vi "ADIS16470 Loop Custom.vi"(8 "error in":errorcluster) -> ()   [LabVIEW 2018]
uses:
  Typedef/ADIS16470 Hardware Configuration.ctl
  <vilib>/Rock Robotics/WPI/SPI/WPI_SPIMode.ctl
  <vilib>/Rock Robotics/SystemInterfaces/DIO/FPGA_DIOChannel.ctl
  <vilib>/Rock Robotics/SystemInterfaces/spilib/spi_bus.ctl
  Typedef/ADIS16470 Process.ctl
  Typedef/ADIS16470 Device Reference.ctl
  Typedef/ADIS16470 Data.ctl
  Typedef/ADIS16470 Status.ctl
  Typedef/ADIS16470 Command Type.ctl
  <vilib>/Rock Robotics/WPI/SPI/WPI_SPIDevRef.ctl
  <vilib>/Rock Robotics/WPI/Interrupt/WPI_InterruptRef.ctl
  <vilib>/Rock Robotics/SystemInterfaces/Interrupt/FPGA_InterruptIndex.ctl
  <vilib>/Rock Robotics/WPI/Encoder/WPI_EncoderDevRef.ctl
  <vilib>/Rock Robotics/SystemInterfaces/Encoder/FPGA_EncoderIdx.ctl
  <vilib>/Rock Robotics/SystemInterfaces/Counter/FPGA_CounterCtrSystemIndex.ctl
  <vilib>/Rock Robotics/WPI/Encoder/WPI_EncoderType.ctl
  <vilib>/Rock Robotics/SystemInterfaces/NetworkCommunication/NetComm_UsageReport_ResourceType.ctl
  Typedef/ADIS16470 Register.ctl
  <vilib>/Rock Robotics/WPI/Counter/WPI_CounterDigitalInputToDigitalSource.vi
  <vilib>/Rock Robotics/SystemInterfaces/CounterEncoderSourceConvertion/FPGA_CounterEncoderSourceConvertionLVSourceTypeToFPGAType.vi
  <vilib>/Rock Robotics/WPI/Interrupt/WPI_InterruptCache.vi
  <vilib>/Rock Robotics/SystemInterfaces/Interrupt/FPGA_InterruptWriteConfiguration.vi
  <vilib>/Rock Robotics/SystemInterfaces/Interrupt/FPGA_WaitOnInterrupt.vi
  <vilib>/Rock Robotics/WPI/Utilities/WPI_UtilitiesTimebaseConstants.vi
  <vilib>/Rock Robotics/SystemInterfaces/Interrupt/FPGA_InterruptReadTimestamp.vi
panel:
  in  "Sychronous Process VI":T1
  in  "Hardware Config":T2={"SPI Clock Rate (Hz)"=2000000.0, "IMU SPI Mode (3)"=enum."Mode 3 (Clk Idle High,Sample on Trailing)", "IMU Reset Pin"=enum."SPI Port CS2", "IMU SPI Bus"=enum."SPI On-Board, CS0", "IMU Data Ready Pin"=enum."SPI Port CS1"}
  out "Waveform Chart":dbl(graph)
  out "Offset Bias":i16[](array[numeric])
  out "xAngle":dbl
  out "yAngle":dbl
  out "Data":dbl[](array[numeric])
  out "Counter":u16
  # "x"
  # "y"
  # "z"
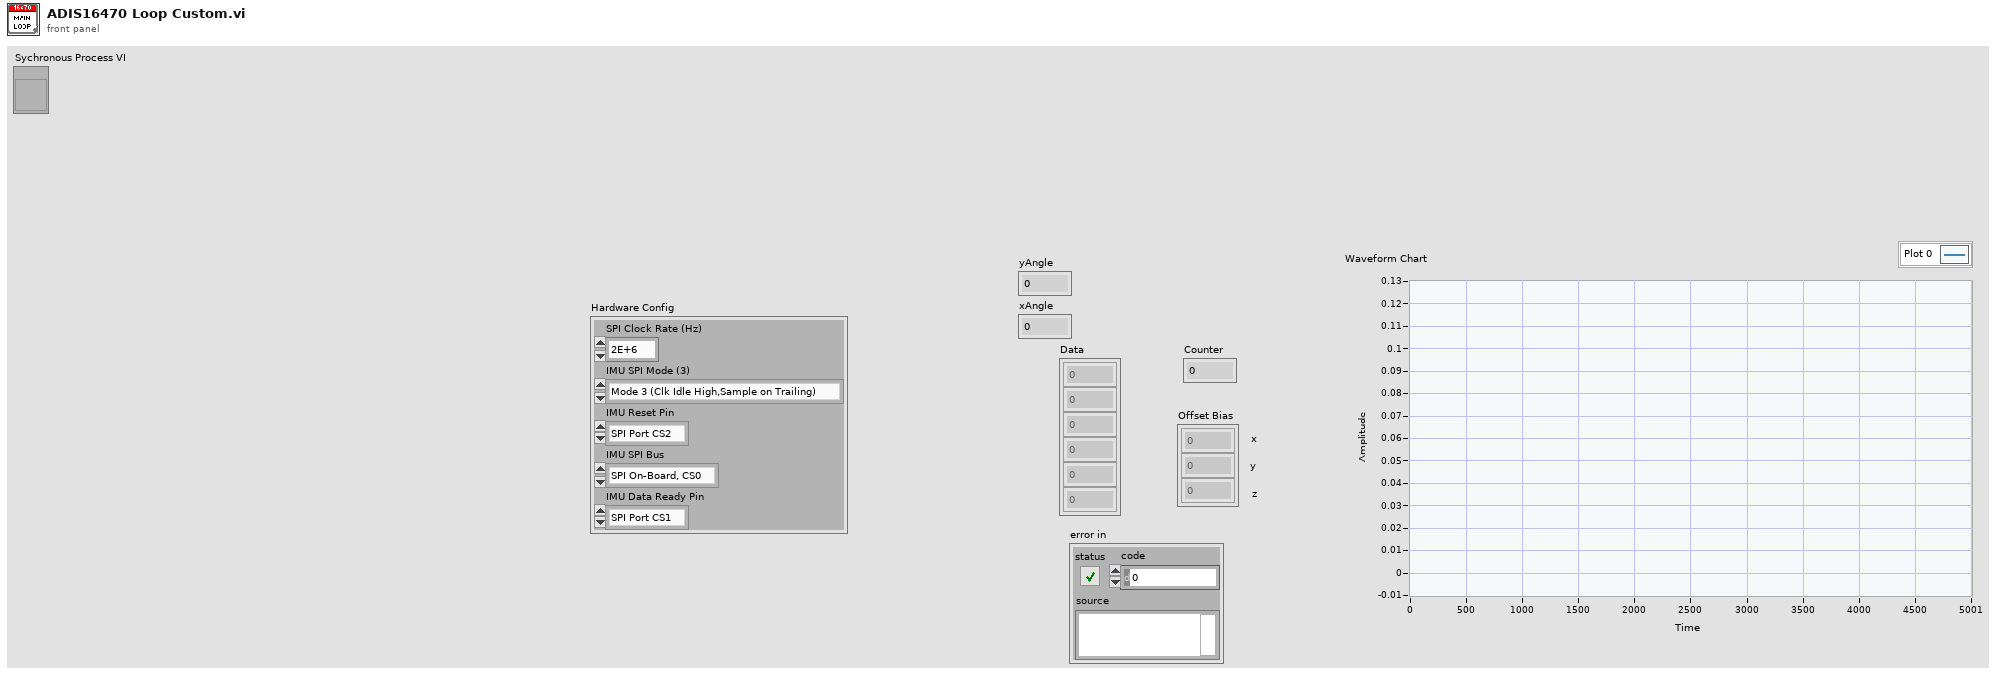
[diagram p1: front panel]
types:
  T1 = typedef "ADIS16470 Process.ctl" = refnum<vi>
  T2 = typedef "ADIS16470 Hardware Configuration.ctl" = cluster{"SPI Clock Rate (Hz)":dbl, "IMU SPI Mode (3)":T3, "IMU Reset Pin":T4, "IMU SPI Bus":T5, "IMU Data Ready Pin":T4}
  T3 = typedef "WPI_SPIMode.ctl" = enum16{"Mode 0 (Clk Idle Low,Sample on Leading)", "Mode 1 (Clk Idle Low,Sample on Trailing)", "Mode 2 (Clk Idle High,Sample on Leading)", "Mode 3 (Clk Idle High,Sample on Trailing)"}
  T4 = typedef "FPGA_DIOChannel.ctl" = enum8{"DIO 0", "DIO 1", "DIO 2", "DIO 3", "DIO 4", "DIO 5", "DIO 6", "DIO 7", "DIO 8", "DIO 9", "DIO MXP 0", "DIO MXP 1", "DIO MXP 2", "DIO MXP 3", "DIO MXP 4", "DIO MXP 5", "DIO MXP 6", "DIO MXP 7", "DIO MXP 8", "DIO MXP 9", "DIO MXP 10", "DIO MXP 11", "DIO MXP 12", "DIO MXP 13", "DIO MXP 14", "DIO MXP 15", "SPI Port CS1", "SPI Port CS2", "SPI Port CS3", "SPI Port MISO", "SPI Port MOSI", "Invalid"}
  T5 = typedef "spi_bus.ctl" = enum16{"SPI On-Board, CS0", "SPI On-Board, CS1", "SPI On-Board, CS2", "SPI On-Board, CS3", "SPI MXP", "Invalid"}
  T6 = typedef "NetComm_UsageReport_ResourceType.ctl" = enum8{"Controller", "Module", "Language", "CANPlugin", "Accelerometer", "ADXL345", "AnalogChannel", "AnalogTrigger", "AnalogTriggerOutput", "CANJaguar", "Compressor", "Counter", "Dashboard", "DigitalInput", "DigitalOutput", "DriverStationCIO", "DriverStationEIO", "DriverStationLCD", "Encoder", "GearTooth", "Gyro", "I2C", "Framework", "Jaguar", "Joystick", "Kinect", "KinectStick", "PIDController", "Preferences", "PWM", "Relay", "RobotDrive", "SerialPort", "Servo", "Solenoid", "SPI", "Task", "Ultrasonic", "Victor", "Button", "Command", "AxisCamera", "PCVideoServer", "SmartDashboard", "Talon", "HiTechnicColorSensor", "HiTechnicAccel", "HiTechnicCompass", "SRF08", "AnalogOutput", "Victor SP", "Talon SRX", "CAN Talon SRX", "ADXL362 Accel", "ADXRS450 Gyro", "Rev SPARK", "Mindsensors SD540", "Digital Filter", "ADIS16448", "PDP", "PCM", "PigeonIMU", "Nidec Brushless", "CTRE CANifier", "CTRE Future 0", "CTRE Future 1", "CTRE Future 2", "CTRE Future 3", "CTRE Future 4", "CTRE Future 5", "CTRE Future 6", "Linear Filter", "Xbox Controller", "USB Camera", "NavX", "Pixy", "Pixy2", "ScanseSweep", "Shuffleboard", "CAN", "Digilent DMC60", "PWM Victor SPX", "Rev SPARK MAX PWM", "Rev SPARK MAX CAN", "ADIS16470"}
  T7 = typedef "ADIS16470 Command Type.ctl" = enum16{"None", "Reset"}
  T8 = typedef "ADIS16470 Device Reference.ctl" = cluster{"DevStatus":errorcluster, "Hardware Config":T2, "End Calibration":refnum<notifier>, "Calibration Complete":refnum<notifier>, "Data FIFO":refnum<k33>, "Status FIFO":refnum<k33>, "Last Value Reference":refnum<data-value>, "Sychronous Process VI":T1, "Cmd FIFO":refnum<k33>}
  T9 = typedef "ADIS16470 Data.ctl" = cluster{"Yaw":dbl, "Timestamp":dbl, "Timestamp Delta":dbl, "Sample Count":u16}
  T10 = typedef "ADIS16470 Status.ctl" = cluster{"Calibrated?":bool}
  T11 = typedef "WPI_SPIDevRef.ctl" = cluster{"DevStatus":errorcluster, "Handle":i32, "SPI Bus":T5}
  T12 = typedef "WPI_InterruptRef.ctl" = cluster{"DevStatus":errorcluster, "InterruptIndex":T13}
  T13 = typedef "FPGA_InterruptIndex.ctl" = enum8{"0", "1", "2", "3", "4", "5", "6", "7", "Invalid"}
  T14 = typedef "WPI_EncoderDevRef.ctl" = cluster{"DevStatus":errorcluster, "EncoderIndex":T15, "CounterIndex":T16, "DistancePerCount":dbl, "Decoding Type":T17}
  T15 = typedef "FPGA_EncoderIdx.ctl" = enum8{"Enc 0", "Enc 1", "Enc 2", "Enc 3", "Enc 4", "Enc 5", "Enc 6", "Enc 7", "Invalid"}
  T16 = typedef "FPGA_CounterCtrSystemIndex.ctl" = enum8{"Ctr 0", "Ctr 1", "Ctr 2", "Ctr 3", "Ctr 4", "Ctr 5", "Ctr 6", "Ctr 7", "Invalid"}
  T17 = typedef "WPI_EncoderType.ctl" = enum16{"1x", "2x", "4x"}
  T18 = cluster{"ADIS16470DevRef":T8, "SPIDevRef":T11, "InterruptRef":T12, "Sensor to Robot Rotation":dbl[][], "Yaw":dbl, "Data Counter":u16, "First Run":bool, "TimeStamp Prev":dbl, "Time Delta":dbl, "Encoder Right":T14, "Encoder Left":T14, "Encoder Data":cluster{"Left Distance":dbl, "Right Distance":dbl}}
  T19 = typedef "ADIS16470 Register.ctl" = u8
  T20 = typedef "WPI_DigitalOutputDevRef.ctl" = cluster{"DIO Channel":T4, "DevStatus":errorcluster}
  T21 = typedef "WPI_DigitalInputDevRef.ctl" = cluster{"DevStatus":errorcluster, "DIO Channel":T4}
  T22 = typedef "FPGA_CounterEncoderSourceConvertionLVSourceType.ctl" = cluster{"DevStatus":errorcluster, "AnalogTriggerMode?":bool, "DigitalMode":cluster{"DIO Channel":T23}, "AnalogTriggerMode":cluster{"AnalogTriggerIndex":T24, "OutputType":T25}}
  T23 = typedef "FPGA_DIODigitalSourceChannel.ctl" = enum8{"DIO 0", "DIO 1", "DIO 2", "DIO 3", "DIO 4", "DIO 5", "DIO 6", "DIO 7", "DIO 8", "DIO 9", "DIO MXP 0", "DIO MXP 1", "DIO MXP 2", "DIO MXP 3", "DIO MXP 4", "DIO MXP 5", "DIO MXP 6", "DIO MXP 7", "DIO MXP 8", "DIO MXP 9", "DIO MXP 10", "DIO MXP 11", "DIO MXP 12", "DIO MXP 13", "DIO MXP 14", "DIO MXP 15", "SPI Port CS1", "SPI Port CS2", "SPI Port CS3", "SPI Port MISO", "SPI Port MOSI", "Disabled"}
  T24 = typedef "FPGA_AnalogTriggerIndex.ctl" = enum8{"Trig 0", "Trig 1", "Trig 2", "Trig 3", "Trig 4", "Trig 5", "Trig 6", "Trig 7", "Invalid"}
  T25 = typedef "FPGA_AnalogTriggerOutType.ctl" = enum16{"InWindow", "TriggerState", "Rising", "Falling"}
  T26 = cluster{"Left Distance":dbl, "Right Distance":dbl}
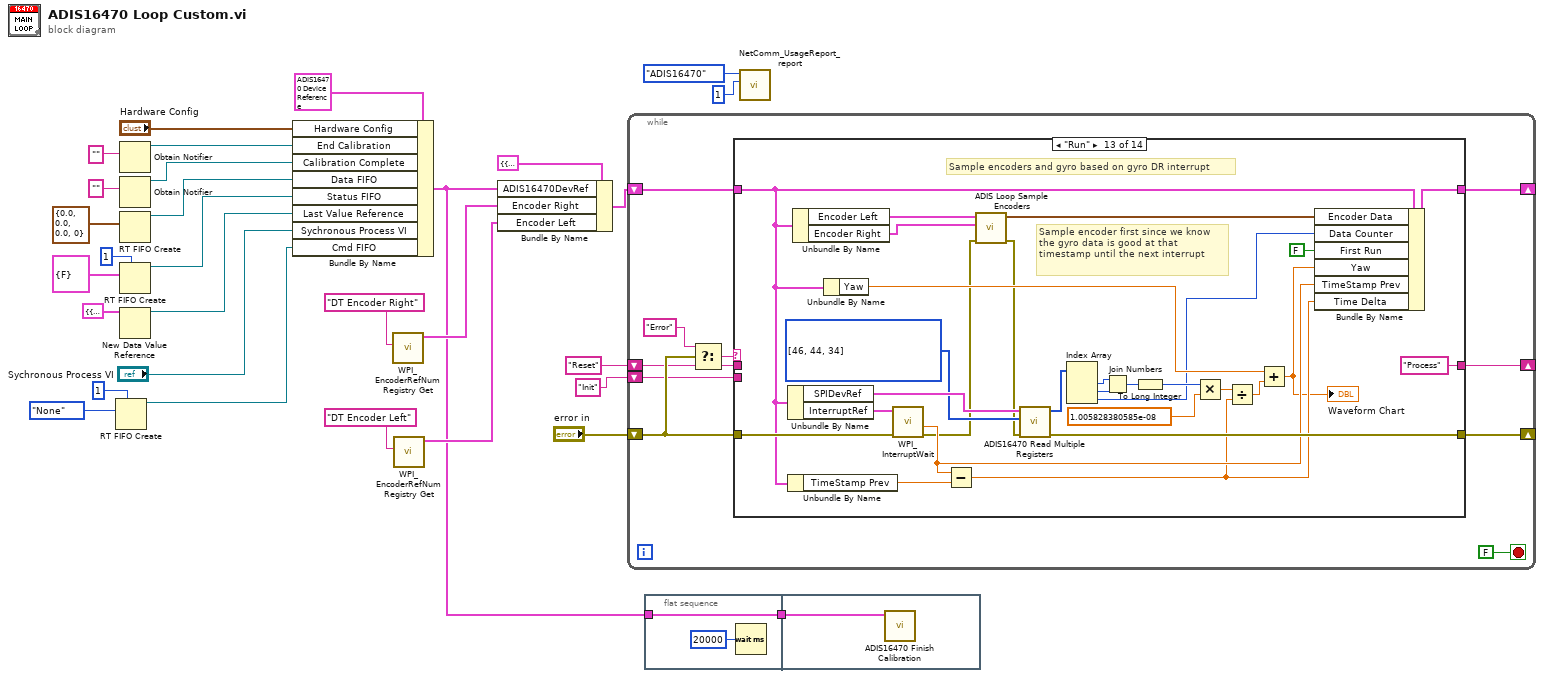
[diagram p0: block diagram]
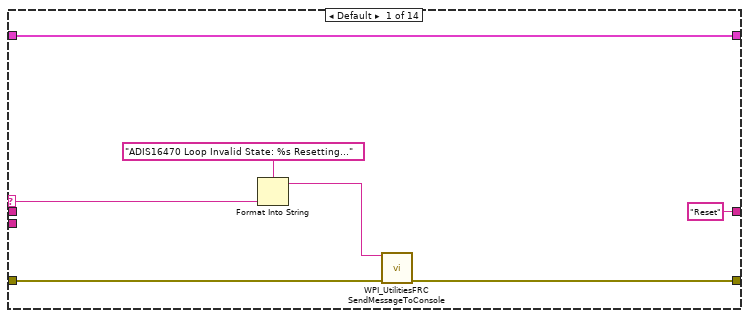
[diagram p2: hidden frame]
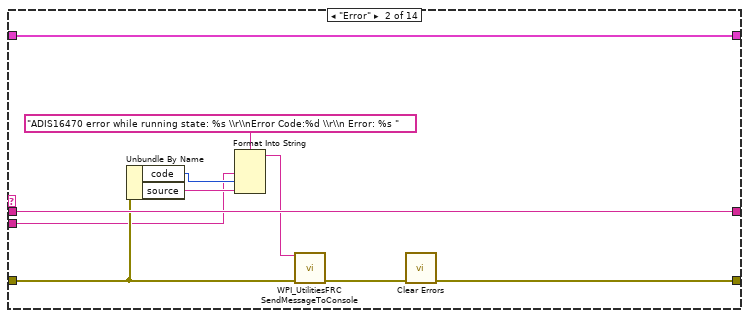
[diagram p3: hidden frame]
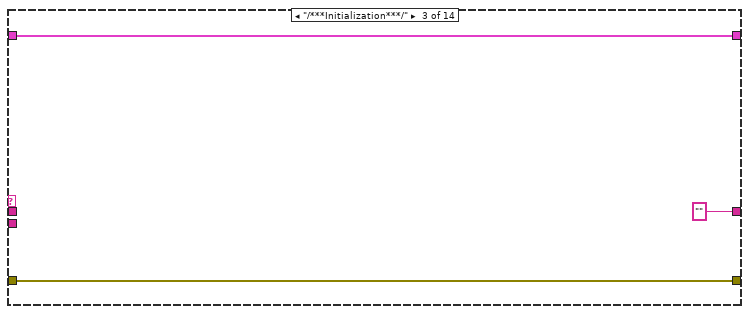
[diagram p4: hidden frame]
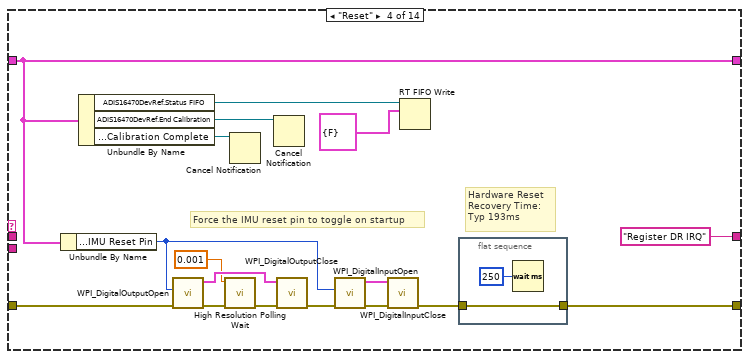
[diagram p5: hidden frame]
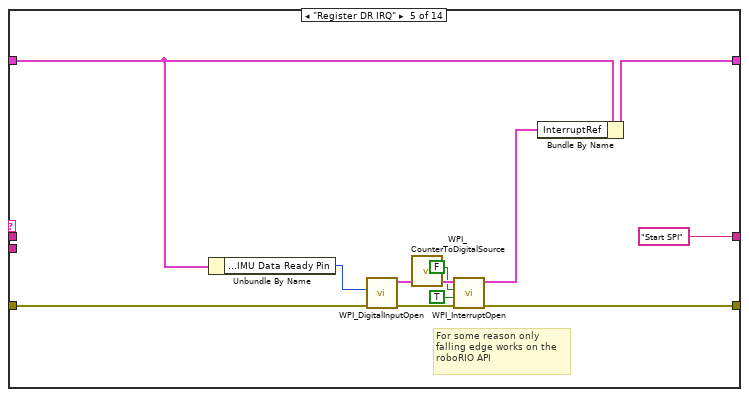
[diagram p6: hidden frame]
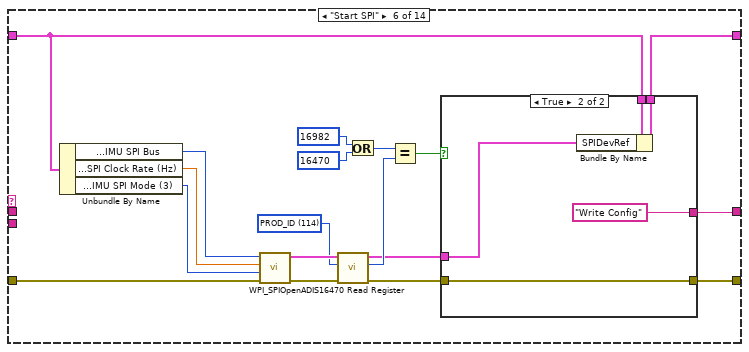
[diagram p7: hidden frame]
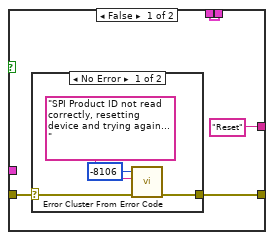
[diagram p8: hidden frame]
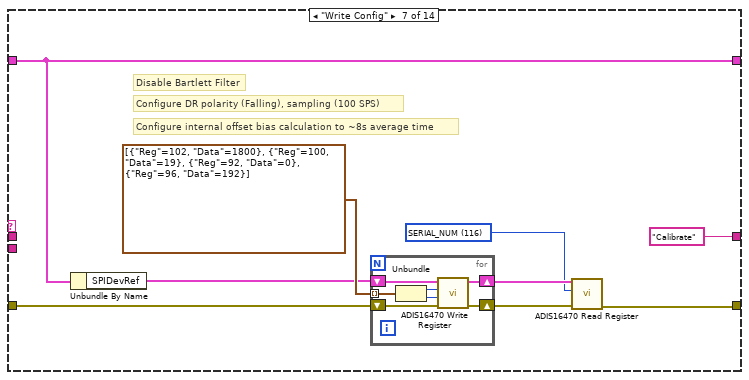
[diagram p10: hidden frame]
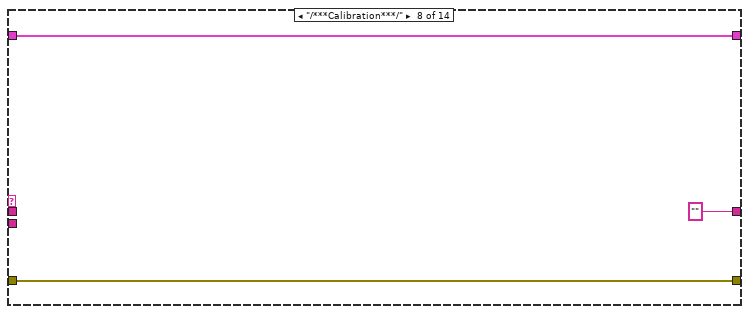
[diagram p11: hidden frame]
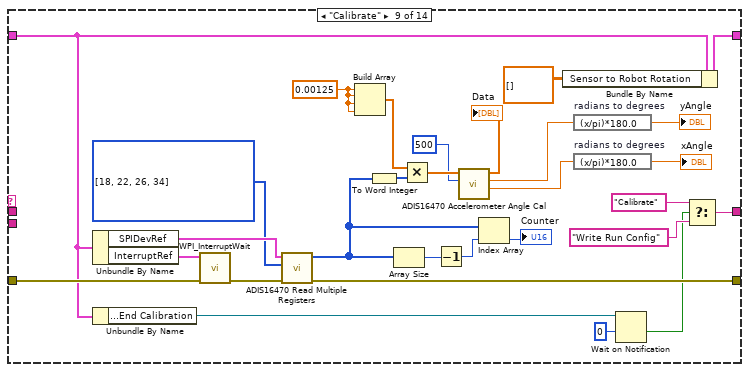
[diagram p12: hidden frame]
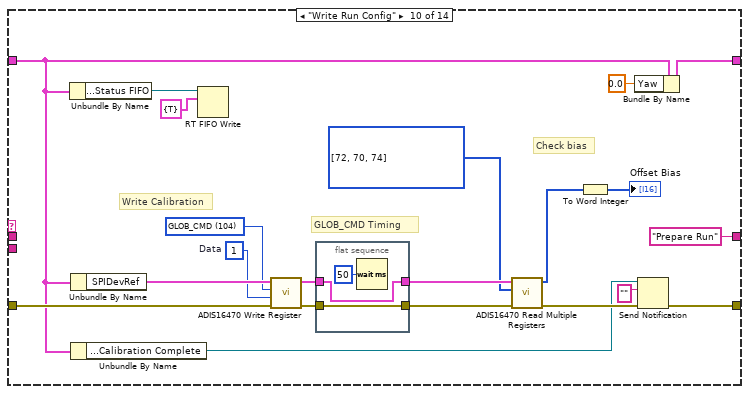
[diagram p13: hidden frame]
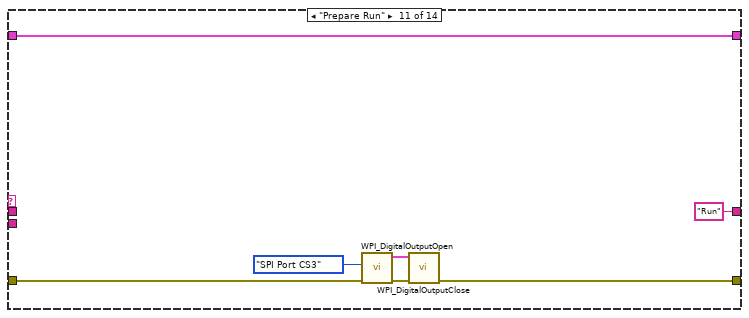
[diagram p14: hidden frame]
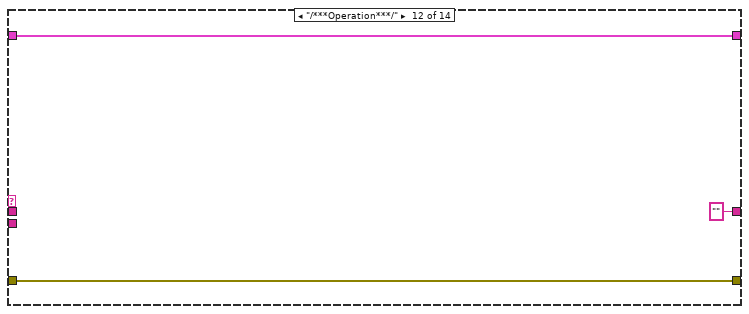
[diagram p15: hidden frame]
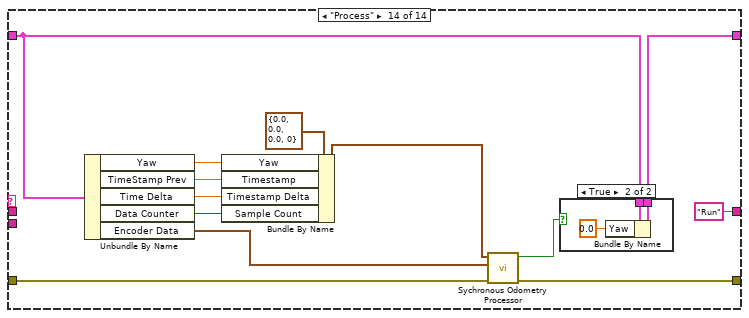
[diagram p16: hidden frame]
diagram:
  n1 = RT FIFO Create(1:ADIS16470_Command_Type."None", 4:u32 1 ("size (10)")) -> (8:w9:refnum<k33>)  [unwired: 6 in, 2 out]
  n2 = Obtain Notifier(notification data type="") -> (notifier out=w22:refnum<notifier>)  [unwired: 3 in, 2 out]
  n3 = Obtain Notifier(notification data type="") -> (notifier out=w23:refnum<notifier>)  [unwired: 3 in, 2 out]
  n4 = RT FIFO Create(1:T9 {"Yaw"=0.0, "Timestamp"=0.0, "Timestamp Delta"=0.0, "Sample Count"=0}) -> (8:w16:refnum<k33>)  [unwired: 7 in, 2 out]
  n5 = RT FIFO Create(1:T10 {"Calibrated?"=FALSE}, 4:u32 1 ("size (10)")) -> (8:w15:refnum<k33>)  [unwired: 6 in, 2 out]
  n6 = New Data Value Reference(data value=cluster{T9, T10} {{"Yaw"=0.0, "Timestamp"=0.0, "Timestamp Delta"=0.0, "Sample Count"=0}, {"Calibrated?"=FALSE}} ("output cluster")) -> (data value reference=w13:refnum<data-value>)  [unwired: 1 in, 1 out]
  n7 = Bundle By Name(cluster=T8 {"DevStatus"={"status"=FALSE, "code"=0, "source"=""}, "Hardware Config"={"SPI Clock Rate (Hz)"=1000000.0, "IMU SPI Mode (3)"=enum."Mode 3 (Clk Idle High,Sample on Trailing)", "IMU Reset Pin"=enum."SPI Port CS2", "IMU SPI Bus"=enum."SPI On-Board, CS0", "IMU Data Ready Pin"=enum."SPI Port CS1"}, "End Calibration"=refnum, "Calibration Complete"=refnum, "Data FIFO"=refnum, "Status FIFO"=refnum, "Last Value Reference"=refnum, "Sychronous Process VI"=refnum, "Cmd FIFO"=refnum} ("ADIS16470DevRef"), "Hardware Config"="Hardware Config", "End Calibration"=w22, "Calibration Complete"=w23, "Data FIFO"=w16, "Status FIFO"=w15, "Last Value Reference"=w13, "Sychronous Process VI"="Sychronous Process VI", "Cmd FIFO"=w9) -> (w2:T8)
  n8 = call <vilib>:"WPI_EncoderRefNum Registry Get.vi"("refnum name"="DT Encoder Right") -> ("EncoderDevRef"=w3:T14)  [unwired: 9 in, 1 out]
  n9 = call <vilib>:"WPI_EncoderRefNum Registry Get.vi"("refnum name"="DT Encoder Left") -> ("EncoderDevRef"=w4:T14)  [unwired: 9 in, 1 out]
  n10 = Bundle By Name(cluster=T18 {"ADIS16470DevRef"={"DevStatus"={"status"=FALSE, "code"=0, "source"=""}, "Hardware Config"={"SPI Clock Rate (Hz)"=1000000.0, "IMU SPI Mode (3)"=enum."Mode 3 (Clk Idle High,Sample on Trailing)", "IMU Reset Pin"=enum."SPI Port CS2", "IMU SPI Bus"=enum."SPI On-Board, CS0", "IMU Data Ready Pin"=enum."SPI Port CS1"}, "End Calibration"=refnum, "Calibration Complete"=refnum, "Data FIFO"=refnum, "Status FIFO"=refnum, "Last Value Reference"=refnum, "Sychronous Process VI"=refnum, "Cmd FIFO"=refnum}, "SPIDevRef"={"DevStatus"={"status"=FALSE, "code"=0, "source"=""}, "Handle"=0, "SPI Bus"=enum."SPI On-Board, CS0"}, "InterruptRef"={"DevStatus"={"status"=FALSE, "code"=0, "source"=""}, "InterruptIndex"=enum."Invalid"}, "Sensor to Robot Rotation"=[[0.0, 0.0, 0.0], [0.0, 0.0, 0.0], [0.0, 0.0, 0.0]], "Yaw"=0.0, "Data Counter"=0, "First Run"=FALSE, "TimeStamp Prev"=0.0, "Time Delta"=0.0, "Encoder Right"={"DevStatus"={"status"=FALSE, "code"=0, "source"=""}, "EncoderIndex"=enum."Invalid", "CounterIndex"=enum."Invalid", "DistancePerCount"=1.0, "Decoding Type"=enum."4x"}, "Encoder Left"={"DevStatus"={"status"=FALSE, "code"=0, "source"=""}, "EncoderIndex"=enum."Invalid", "CounterIndex"=enum."Invalid", "DistancePerCount"=1.0, "Decoding Type"=enum."4x"}, "Encoder Data"={"Left Distance"=0.0, "Right Distance"=0.0}}, "ADIS16470DevRef"=w2, "Encoder Right"=w3, "Encoder Left"=w4) -> (w28:T18)
  n11 = while {
    shift-right: [w36] -> _
    shift-left: "Reset" -> [w33]
    shift-right: [w38] -> _
    shift-left: w28 -> [w39]
    shift-right: [w37] -> _
    shift-left: "error in" -> [w35]
    shift-left: "Init" -> [w31]
    stop <- FALSE stop-if-true
    n12 = Select(t="Error", s=w35, f=w33) -> (s? t:f=w34:string)
    n13 = case shown="\"Run\"" w34 {
      selector: w34 -> [w46 _ _ _ _ _ _ _ _ _ _ _ _ _]
      tunnel: w39 -> [w47 w57 w60 w65 w83 w99 w131 w142 w155 w176 w202 w205 w212 w245]
      tunnel: [w47 w57 w60 w65 w90 w100 w131 w142 w157 w183 w202 w205 w223 w235] -> w38
      tunnel: w35 -> [w45 w53 w59 w72 w86 w106 w128 w141 w170 w190 w198 w204 w231 w239]
      tunnel: [w44 w54 w59 w67 w89 w98 w125 w141 w167 w178 w197 w204 w229 w238] -> w37
      tunnel: ["Reset" w56 "" "Register DR IRQ" "Start SPI" w101 "Calibrate" "" w154 "Prepare Run" "Run" "" "Process" "Run"] -> w36
      tunnel: w33 -> [_ w56 _ _ _ _ _ _ _ _ _ _ _ _]
      tunnel: w31 -> [_ w48 _ _ _ _ _ _ _ _ _ _ _ _]
      frame Default {
        n14 = Format Into String(format string="ADIS16470 Loop Invalid State: %s Resetting...", w46) -> (resulting string=w43:string)  [unwired: 2 in, 1 out]
        n15 = call <vilib>:"WPI_UtilitiesFRC SendMessageToConsole.vi"("Message"=w43, "error in (no error)"=w45) -> ("error out"=w44:errorcluster)  [unwired: 13 in]
      }
      frame "Error" {
        n16 = Unbundle By Name(w53) -> ("code"=w50:i32, "source"=w49:string)
        n17 = Format Into String(format string="ADIS16470 error while running state: %s \\r\\nError Code:%d \\r\\n Error: %s ", w48, w50, w49) -> (resulting string=w52:string)  [unwired: 2 in, 1 out]
        n18 = call <vilib>:"WPI_UtilitiesFRC SendMessageToConsole.vi"("Message"=w52, "error in (no error)"=w53) -> ("error out"=w55:errorcluster)  [unwired: 13 in]
        n19 = call <vilib>:"Clear Errors.vi"("error in (no error)"=w55) -> ("error out"=w54:errorcluster)  [unwired: 5 in, 1 out]
      }
      frame "/***Initialization***/" {
      }
      frame "Reset" {
        # "Hardware Reset Recovery Time: Typ 193ms"
        # "Force the IMU reset pin to toggle on startup"
        n20 = Unbundle By Name(w65) -> ("ADIS16470DevRef.Hardware Config.IMU Reset Pin"=w73:T4)
        n21 = Unbundle By Name(w65) -> ("ADIS16470DevRef.Status FIFO"=w62:refnum<k33>, "ADIS16470DevRef.End Calibration"=w63:refnum<notifier>, "ADIS16470DevRef.Calibration Complete"=w64:refnum<notifier>)
        n22 = call <vilib>:"WPI_DigitalOutputOpen.vi"("error in (no error)"=w72, "DIO Channel"=w73) -> ("error out"=w70:errorcluster, "DigitalOutputDevRef"=w74:T20)  [unwired: 8 in]
        n23 = call <vilib>:"High Resolution Polling Wait.vi"("error in (no error)"=w70, "seconds to wait"=0.001) -> ("error out"=w69:errorcluster)  [unwired: 9 in]
        n24 = Cancel Notification(0:w64) -> ()  [unwired: 1 in, 3 out]
        n25 = Cancel Notification(0:w63) -> ()  [unwired: 1 in, 3 out]
        n26 = call <vilib>:"WPI_DigitalOutputClose.vi"("error in (no error)"=w69, "DigitalOutputDevRef"=w74) -> ("error out"=w77:errorcluster)  [unwired: 9 in]
        n27 = call <vilib>:"WPI_DigitalInputOpen.vi"("error in (no error)"=w77, "DIO Channel"=w73) -> ("error out"=w76:errorcluster, "DigitalInputDevRef"=w75:T21)  [unwired: 8 in]
        n28 = call <vilib>:"WPI_DigitalInputClose.vi"("error in (no error)"=w76, "DigitalInputDevRef"=w75) -> ("error out"=w66:errorcluster)  [unwired: 9 in]
        n29 = RT FIFO Write(0:w62, 1:T10 {"Calibrated?"=FALSE} ("element")) -> ()  [unwired: 3 in, 4 out]
        n30 = flat-sequence {
          tunnel: [w79] -> w67
          tunnel: w66 -> [w79]
          frame #0 {
            n31 = Wait (ms)(milliseconds to wait=u32 250) -> ()  [unwired: 1 out]
          }
        }
      }
      frame "Register DR IRQ" {
        # "For some reason only\nfalling edge works on the\nroboRIO API"
        n32 = Unbundle By Name(w83) -> ("ADIS16470DevRef.Hardware Config.IMU Data Ready Pin"=w82:T4)
        n33 = call <vilib>:"WPI_DigitalInputOpen.vi"("error in (no error)"=w86, "DIO Channel"=w82) -> ("error out"=w85:errorcluster, "DigitalInputDevRef"=w84:T21)  [unwired: 8 in]
        n34 = call-poly <vilib>:"WPI_CounterToDigitalSource.vi"("DigitalInputDevRef"=w84) -> ("Digital Source"=w87:T22)  [unwired: 6 in]
        n35 = call <vilib>:"WPI_InterruptOpen.vi"("error in (no error)"=w85, "Falling Edge"=TRUE, "Rising Edge"=FALSE, "Source"=w87) -> ("error out"=w89:errorcluster, "InterruptRef"=w88:T12)  [unwired: 6 in]
        n36 = Bundle By Name(cluster=w83, "InterruptRef"=w88) -> (w90:T18)
      }
      frame "Start SPI" {
        w93 = T19 114 items=["Reserved1"=0, "DIAG_STAT"=2, "X_GYRO_LOW"=4, "X_GYRO_OUT"=6, "Y_GYRO_LOW"=8, "Y_GYRO_OUT"=10, "Z_GYRO_LOW"=12, "Z_GYRO_OUT"=14, "X_ACCL_LOW"=16, "X_ACCL_OUT"=18, "Y_ACCL_LOW"=20, "Y_ACCL_OUT"=22, "Z_ACCL_LOW"=24, "Z_ACCL_OUT"=26, "TEMP_OUT"=28, "TIME_STAMP"=30, "Reseved2"=32, "DATA_CNTR"=34, "X_DELTANG_LOW"=36, "X_DELTANG_OUT"=38, "Y_DELTANG_LOW"=40, "Y_DELTANG_OUT"=42, "Z_DELTANG_LOW"=44, "Z_DELTANG_OUT"=46, "X_DELTVEL_LOW"=48, "X_DELTVEL_OUT"=50, "Y_DELTVEL_LOW"=52, "Y_DELTVEL_OUT"=54, "Z_DELTVEL_LOW"=56, "Z_DELTVEL_OUT"=58, "Reserved3"=60, "Reserved4"=62, "XG_BIAS_LOW"=64, "XG_BIAS_HIGH"=66, "YG_BIAS_LOW"=68, "YG_BIAS_OUT"=70, "ZG_BIAS_LOW"=72, "ZG_BIAS_OUT"=74, "XA_BIAS_LOW"=76, "XA_BIAS_HIGH"=78, "YA_BIAS_LOW"=80, "YA_BIAS_OUT"=82, "ZA_BIAS_LOW"=84, "ZA_BIAS_OUT"=86, "Reserved5"=88, "Reserved6"=90, "FILT_CTRL"=92, "Reserved5"=94, "MSC_CTRL"=96, "UP_SCALE"=98, "DEC_RATE"=100, "NULL_CNFG"=102, "GLOB_CMD"=104, "Reserved6"=106, "FIRM_REV"=108, "FIRM_DM"=110, "FIRM_Y"=112, "PROD_ID"=114, "SERIAL_NUM"=116, "USER_SCR1"=118, "USER_SCR2"=120, "USER_SCR3"=122, "FLSHCNT_LOW"=124, "FLSHCNT_HIGH"=126] ("ADIS16448 Register")
        n37 = Unbundle By Name(w99) -> ("ADIS16470DevRef.Hardware Config.IMU SPI Bus"=w102:T5, "ADIS16470DevRef.Hardware Config.SPI Clock Rate (Hz)"=w103:dbl, "ADIS16470DevRef.Hardware Config.IMU SPI Mode (3)"=w104:T3)
        n38 = call <vilib>:"WPI_SPIOpen.vi"("error in"=w106, "Mode (3)"=w104, "Clock Rate (Hz)"=w103, "SPI Bus"=w102) -> ("error out"=w95:errorcluster, "SPIDevRef"=w94:T11)  [unwired: 6 in]
        n39 = call "ADIS16470 Read Register.vi"("error in (no error)"=w95, "ADIS16470 Register"=w93, "SPIDevRef in"=w94) -> ("error out"=w96:errorcluster, "Register Value"=w97:u16, "SPIDevRef out"=w92:T11)  [unwired: 6 in]
        n40 = Or(x=u16 16982 ("y"), y=u16 16470) -> (x .or. y?=w107:u16)
        n41 = Equal?(x=w107, y=w97) -> (x = y?=w105:bool)
        n42 = case shown="True" w105 {
          tunnel: ["Reset" "Write Config"] -> w101
          tunnel: w99 -> [w112 w122]
          tunnel: [w112 w121] -> w100
          tunnel: [w111 w119] -> w98
          tunnel: w96 -> [w110 w119]
          tunnel: w92 -> [_ w120]
          frame False {
            n43 = case shown="No Error" w110 {
              selector: w110 -> [w116 w118]
              tunnel: [w117 w118] -> w111
              frame No Error {
                n44 = call <vilib>:"Error Cluster From Error Code.vi"("error in (no error)"=w116, "error message (\"\")"="SPI Product ID not read correctly, resetting device and trying again..." ("error message (\"\")"), "error code (0)"=-8106) -> ("error out"=w117:errorcluster)  [unwired: 6 in]
              }
              frame Error {
              }
            }
          }
          frame True {
            n45 = Bundle By Name(cluster=w122, "SPIDevRef"=w120) -> (w121:T18)
          }
        }
      }
      frame "Write Config" {
        w124 = T19 116 items=["Reserved1"=0, "DIAG_STAT"=2, "X_GYRO_LOW"=4, "X_GYRO_OUT"=6, "Y_GYRO_LOW"=8, "Y_GYRO_OUT"=10, "Z_GYRO_LOW"=12, "Z_GYRO_OUT"=14, "X_ACCL_LOW"=16, "X_ACCL_OUT"=18, "Y_ACCL_LOW"=20, "Y_ACCL_OUT"=22, "Z_ACCL_LOW"=24, "Z_ACCL_OUT"=26, "TEMP_OUT"=28, "TIME_STAMP"=30, "Reseved2"=32, "DATA_CNTR"=34, "X_DELTANG_LOW"=36, "X_DELTANG_OUT"=38, "Y_DELTANG_LOW"=40, "Y_DELTANG_OUT"=42, "Z_DELTANG_LOW"=44, "Z_DELTANG_OUT"=46, "X_DELTVEL_LOW"=48, "X_DELTVEL_OUT"=50, "Y_DELTVEL_LOW"=52, "Y_DELTVEL_OUT"=54, "Z_DELTVEL_LOW"=56, "Z_DELTVEL_OUT"=58, "Reserved3"=60, "Reserved4"=62, "XG_BIAS_LOW"=64, "XG_BIAS_HIGH"=66, "YG_BIAS_LOW"=68, "YG_BIAS_OUT"=70, "ZG_BIAS_LOW"=72, "ZG_BIAS_OUT"=74, "XA_BIAS_LOW"=76, "XA_BIAS_HIGH"=78, "YA_BIAS_LOW"=80, "YA_BIAS_OUT"=82, "ZA_BIAS_LOW"=84, "ZA_BIAS_OUT"=86, "Reserved5"=88, "Reserved6"=90, "FILT_CTRL"=92, "Reserved5"=94, "MSC_CTRL"=96, "UP_SCALE"=98, "DEC_RATE"=100, "NULL_CNFG"=102, "GLOB_CMD"=104, "Reserved6"=106, "FIRM_REV"=108, "FIRM_DM"=110, "FIRM_Y"=112, "PROD_ID"=114, "SERIAL_NUM"=116, "USER_SCR1"=118, "USER_SCR2"=120, "USER_SCR3"=122, "FLSHCNT_LOW"=124, "FLSHCNT_HIGH"=126] ("ADIS16448 Register")
        # "Configure internal offset bias calculation to ~8s average time"
        # "Configure DR polarity (Falling), sampling (100 SPS)"
        # "Disable Bartlett Filter"
        n46 = Unbundle By Name(w131) -> ("SPIDevRef"=w129:T11)
        n47 = for {
          tunnel: cluster{"Reg":T19, "Data":u16}[] [{"Reg"=102, "Data"=1800}, {"Reg"=100, "Data"=19}, {"Reg"=92, "Data"=0}, {"Reg"=96, "Data"=192}] -> [w139] mode=indexing
          shift-right: [w135] -> w126
          shift-left: w128 -> [w134]
          shift-right: [w133] -> w127
          shift-left: w129 -> [w136]
          n48 = Unbundle(w139) -> ("Reg"=w138:T19, "Data"=w137:u16)
          n49 = call "ADIS16470 Write Register.vi"("error in (no error)"=w134, "Data"=w137, "Register"=w138, "SPIDevRef in"=w136) -> ("error out"=w135:errorcluster, "SPIDevRef out"=w133:T11)  [unwired: 6 in]
        }
        n50 = call "ADIS16470 Read Register.vi"("error in (no error)"=w126, "ADIS16470 Register"=w124, "SPIDevRef in"=w127) -> ("error out"=w125:errorcluster)  [unwired: 6 in, 2 out]
      }
      frame "/***Calibration***/" {
      }
      frame "Calibrate" {
        w161 = 0.00125
        w162 = T19[] [18, 22, 26, 34] items=["Reserved1"=0, "DIAG_STAT"=2, "X_GYRO_LOW"=4, "X_GYRO_OUT"=6, "Y_GYRO_LOW"=8, "Y_GYRO_OUT"=10, "Z_GYRO_LOW"=12, "Z_GYRO_OUT"=14, "X_ACCL_LOW"=16, "X_ACCL_OUT"=18, "Y_ACCL_LOW"=20, "Y_ACCL_OUT"=22, "Z_ACCL_LOW"=24, "Z_ACCL_OUT"=26, "TEMP_OUT"=28, "TIME_STAMP"=30, "Reseved2"=32, "DATA_CNTR"=34, "X_DELTANG_LOW"=36, "X_DELTANG_OUT"=38, "Y_DELTANG_LOW"=40, "Y_DELTANG_OUT"=42, "Z_DELTANG_LOW"=44, "Z_DELTANG_OUT"=46, "X_DELTVEL_LOW"=48, "X_DELTVEL_OUT"=50, "Y_DELTVEL_LOW"=52, "Y_DELTVEL_OUT"=54, "Z_DELTVEL_LOW"=56, "Z_DELTVEL_OUT"=58, "Reserved3"=60, "Reserved4"=62, "XG_BIAS_LOW"=64, "XG_BIAS_HIGH"=66, "YG_BIAS_LOW"=68, "YG_BIAS_OUT"=70, "ZG_BIAS_LOW"=72, "ZG_BIAS_OUT"=74, "XA_BIAS_LOW"=76, "XA_BIAS_HIGH"=78, "YA_BIAS_LOW"=80, "YA_BIAS_OUT"=82, "ZA_BIAS_LOW"=84, "ZA_BIAS_OUT"=86, "Reserved5"=88, "Reserved6"=90, "FILT_CTRL"=92, "Reserved5"=94, "MSC_CTRL"=96, "UP_SCALE"=98, "DEC_RATE"=100] ("Registers")
        n51 = Unbundle By Name(w155) -> ("SPIDevRef"=w168:T11, "InterruptRef"=w171:T12)
        n52 = Unbundle By Name(w155) -> ("ADIS16470DevRef.End Calibration"=w145:refnum<notifier>)
        n53 = call <vilib>:"WPI_InterruptWait.vi"("error in (no error)"=w170, "InterruptRef"=w171) -> ("error out"=w169:errorcluster)  [unwired: 5 in, 4 out]
        n54 = call "ADIS16470 Read Multiple Registers.vi"("error in (no error)"=w169, "Registers"=w162, "SPIDevRef"=w168) -> ("error out"=w167:errorcluster, "Values"=w150:u16[])  [unwired: 7 in]
        n55 = Build Array(w161, w161, w161, w161) -> (w166:dbl[])
        n56 = To Word Integer(number=w150) -> (16bit integer=w151:i16[])
        n57 = Array Size(array=w150) -> (size(s)=w165:i32)
        n58 = Multiply(x=w166, y=w151) -> (x*y=w160:dbl[])
        n59 = Decrement(x=w165) -> (x-1=w164:i32)
        n60 = call "ADIS16470 Accelerometer Angle Cal.vi"("average samples"=500, "Raw Accel In"=w160) -> ("xAngle"=w148:dbl, "yAngle"=w147:dbl, "Average Accel Out"=→"Data":dbl[])  [unwired: 7 in]
        n61 = Index Array(array=w150, index=w164) -> (element=→"Counter":u16)
        n62 = Bundle By Name(cluster=w155, "Sensor to Robot Rotation"=dbl[][] []) -> (w157:T18)
        n63 = expression code="(x/pi)*180.0" "radians to degrees"(w147) -> (→"yAngle":dbl)
        n64 = expression code="(x/pi)*180.0" "radians to degrees"(w148) -> (→"xAngle":dbl)
        n65 = Wait on Notification(notifier=w145, timeout in ms (-1)=0) -> (timed out?=w143:bool)  [unwired: 2 in, 3 out]
        n66 = Select(t="Calibrate", s=w143, f="Write Run Config") -> (s? t:f=w154:string)
      }
      frame "Write Run Config" {
        w173 = T19 104 items=["Reserved1"=0, "DIAG_STAT"=2, "X_GYRO_LOW"=4, "X_GYRO_OUT"=6, "Y_GYRO_LOW"=8, "Y_GYRO_OUT"=10, "Z_GYRO_LOW"=12, "Z_GYRO_OUT"=14, "X_ACCL_LOW"=16, "X_ACCL_OUT"=18, "Y_ACCL_LOW"=20, "Y_ACCL_OUT"=22, "Z_ACCL_LOW"=24, "Z_ACCL_OUT"=26, "TEMP_OUT"=28, "TIME_STAMP"=30, "Reseved2"=32, "DATA_CNTR"=34, "X_DELTANG_LOW"=36, "X_DELTANG_OUT"=38, "Y_DELTANG_LOW"=40, "Y_DELTANG_OUT"=42, "Z_DELTANG_LOW"=44, "Z_DELTANG_OUT"=46, "X_DELTVEL_LOW"=48, "X_DELTVEL_OUT"=50, "Y_DELTVEL_LOW"=52, "Y_DELTVEL_OUT"=54, "Z_DELTVEL_LOW"=56, "Z_DELTVEL_OUT"=58, "Reserved3"=60, "Reserved4"=62, "XG_BIAS_LOW"=64, "XG_BIAS_HIGH"=66, "YG_BIAS_LOW"=68, "YG_BIAS_OUT"=70, "ZG_BIAS_LOW"=72, "ZG_BIAS_OUT"=74, "XA_BIAS_LOW"=76, "XA_BIAS_HIGH"=78, "YA_BIAS_LOW"=80, "YA_BIAS_OUT"=82, "ZA_BIAS_LOW"=84, "ZA_BIAS_OUT"=86, "Reserved5"=88, "Reserved6"=90, "FILT_CTRL"=92, "Reserved5"=94, "MSC_CTRL"=96, "UP_SCALE"=98, "DEC_RATE"=100, "NULL_CNFG"=102, "GLOB_CMD"=104, "Reserved6"=106, "FIRM_REV"=108, "FIRM_DM"=110, "FIRM_Y"=112, "PROD_ID"=114, "SERIAL_NUM"=116, "USER_SCR1"=118, "USER_SCR2"=120, "USER_SCR3"=122, "FLSHCNT_LOW"=124, "FLSHCNT_HIGH"=126] ("Register")
        w189 = u16 1  # Data
        w184 = T19[] [72, 70, 74] items=["Reserved1"=0, "DIAG_STAT"=2, "X_GYRO_LOW"=4, "X_GYRO_OUT"=6, "Y_GYRO_LOW"=8, "Y_GYRO_OUT"=10, "Z_GYRO_LOW"=12, "Z_GYRO_OUT"=14, "X_ACCL_LOW"=16, "X_ACCL_OUT"=18, "Y_ACCL_LOW"=20, "Y_ACCL_OUT"=22, "Z_ACCL_LOW"=24, "Z_ACCL_OUT"=26, "TEMP_OUT"=28, "TIME_STAMP"=30, "Reseved2"=32, "DATA_CNTR"=34, "X_DELTANG_LOW"=36, "X_DELTANG_OUT"=38, "Y_DELTANG_LOW"=40, "Y_DELTANG_OUT"=42, "Z_DELTANG_LOW"=44, "Z_DELTANG_OUT"=46, "X_DELTVEL_LOW"=48, "X_DELTVEL_OUT"=50, "Y_DELTVEL_LOW"=52, "Y_DELTVEL_OUT"=54, "Z_DELTVEL_LOW"=56, "Z_DELTVEL_OUT"=58, "Reserved3"=60, "Reserved4"=62, "XG_BIAS_LOW"=64, "XG_BIAS_HIGH"=66, "YG_BIAS_LOW"=68, "YG_BIAS_OUT"=70, "ZG_BIAS_LOW"=72, "ZG_BIAS_OUT"=74, "XA_BIAS_LOW"=76, "XA_BIAS_HIGH"=78, "YA_BIAS_LOW"=80, "YA_BIAS_OUT"=82, "ZA_BIAS_LOW"=84, "ZA_BIAS_OUT"=86, "Reserved5"=88, "Reserved6"=90, "FILT_CTRL"=92, "Reserved5"=94, "MSC_CTRL"=96, "UP_SCALE"=98, "DEC_RATE"=100] ("Registers")
        # "Write Calibration"
        # "GLOB_CMD Timing"
        # "Check bias"
        n67 = Unbundle By Name(w176) -> ("ADIS16470DevRef.Status FIFO"=w175:refnum<k33>)
        n68 = Unbundle By Name(w176) -> ("SPIDevRef"=w191:T11)
        n69 = Unbundle By Name(w176) -> ("ADIS16470DevRef.Calibration Complete"=w179:refnum<notifier>)
        n70 = RT FIFO Write(0:w175, 1:T10 {"Calibrated?"=TRUE} ("element")) -> ()  [unwired: 3 in, 4 out]
        n71 = call "ADIS16470 Write Register.vi"("error in (no error)"=w190, "Data"=w189, "Register"=w173, "SPIDevRef in"=w191) -> ("error out"=w188:errorcluster, "SPIDevRef out"=w187:T11)  [unwired: 6 in]
        n72 = flat-sequence {
          tunnel: w188 -> [w195]
          tunnel: [w195] -> w186
          tunnel: w187 -> [w193]
          tunnel: [w193] -> w185
          frame #0 {
            n73 = Wait (ms)(milliseconds to wait=u32 50) -> ()  [unwired: 1 out]
          }
        }
        n74 = call "ADIS16470 Read Multiple Registers.vi"("error in (no error)"=w186, "Registers"=w184, "SPIDevRef"=w185) -> ("error out"=w180:errorcluster, "Values"=w182:u16[])  [unwired: 7 in]
        n75 = To Word Integer(number=w182) -> (16bit integer=→"Offset Bias":i16[])
        n76 = Bundle By Name(cluster=w176, "Yaw"=0.0) -> (w183:T18)
        n77 = Send Notification(notification="", notifier=w179, error in (no error)=w180) -> (error out=w178:errorcluster)  [unwired: 1 out]
      }
      frame "Prepare Run" {
        n78 = call <vilib>:"WPI_DigitalOutputOpen.vi"("error in (no error)"=w198, "DIO Channel"=FPGA_DIOChannel."SPI Port CS3") -> ("error out"=w200:errorcluster, "DigitalOutputDevRef"=w201:T20)  [unwired: 8 in]
        n79 = call <vilib>:"WPI_DigitalOutputClose.vi"("error in (no error)"=w200, "DigitalOutputDevRef"=w201) -> ("error out"=w197:errorcluster)  [unwired: 9 in]
      }
      frame "/***Operation***/" {
      }
      frame "Run" {
        w228 = T19[] [46, 44, 34] items=["Reserved1"=0, "DIAG_STAT"=2, "X_GYRO_LOW"=4, "X_GYRO_OUT"=6, "Y_GYRO_LOW"=8, "Y_GYRO_OUT"=10, "Z_GYRO_LOW"=12, "Z_GYRO_OUT"=14, "X_ACCL_LOW"=16, "X_ACCL_OUT"=18, "Y_ACCL_LOW"=20, "Y_ACCL_OUT"=22, "Z_ACCL_LOW"=24, "Z_ACCL_OUT"=26, "TEMP_OUT"=28, "TIME_STAMP"=30, "Reseved2"=32, "DATA_CNTR"=34, "X_DELTANG_LOW"=36, "X_DELTANG_OUT"=38, "Y_DELTANG_LOW"=40, "Y_DELTANG_OUT"=42, "Z_DELTANG_LOW"=44, "Z_DELTANG_OUT"=46, "X_DELTVEL_LOW"=48, "X_DELTVEL_OUT"=50, "Y_DELTVEL_LOW"=52, "Y_DELTVEL_OUT"=54, "Z_DELTVEL_LOW"=56, "Z_DELTVEL_OUT"=58, "Reserved3"=60, "Reserved4"=62, "XG_BIAS_LOW"=64, "XG_BIAS_HIGH"=66, "YG_BIAS_LOW"=68, "YG_BIAS_OUT"=70, "ZG_BIAS_LOW"=72, "ZG_BIAS_OUT"=74, "XA_BIAS_LOW"=76, "XA_BIAS_HIGH"=78, "YA_BIAS_LOW"=80, "YA_BIAS_OUT"=82, "ZA_BIAS_LOW"=84, "ZA_BIAS_OUT"=86, "Reserved5"=88, "Reserved6"=90, "FILT_CTRL"=92, "Reserved5"=94, "MSC_CTRL"=96, "UP_SCALE"=98, "DEC_RATE"=100] ("Registers")
        # "Sample encoder first since we know the gyro data is good at that timestamp until the next interrupt"
        # "Sample encoders and gyro based on gyro DR interrupt"
        n80 = Unbundle By Name(w212) -> ("SPIDevRef"=w230:T11, "InterruptRef"=w232:T12)
        n81 = Unbundle By Name(w212) -> ("TimeStamp Prev"=w218:dbl)
        n82 = Unbundle By Name(w212) -> ("Encoder Left"=w211:T14, "Encoder Right"=w210:T14)
        n83 = Unbundle By Name(w212) -> ("Yaw"=w219:dbl)
        n84 = call <vilib>:"WPI_InterruptWait.vi"("error in (no error)"=w231, "InterruptRef"=w232) -> ("error out"=w213:errorcluster, "TimeStamp"=w217:dbl)  [unwired: 5 in, 3 out]
        n85 = Subtract(x=w217, y=w218) -> (x-y=w214:dbl)
        n86 = call "ADIS Loop Sample Encoders.vi"("error in (no error)"=w213, "Right Encoder"=w210, "Left Encoder"=w211) -> ("error out"=w207:errorcluster, "cluster"=w209:T26)  [unwired: 7 in]
        n87 = call "ADIS16470 Read Multiple Registers.vi"("error in (no error)"=w207, "Registers"=w228, "SPIDevRef"=w230) -> ("error out"=w229:errorcluster, "Values"=w227:u16[])  [unwired: 7 in]
        n88 = Index Array(array=w227) -> (element #1=w226:u16, element #2=w225:u16, element #3=w206:u16)  [unwired: 3 in]
        n89 = Join Numbers(hi=w226, lo=w225) -> ((hi.lo)=w216:u32)
        n90 = To Long Integer(number=w216) -> (32bit integer=w215:i32)
        n91 = Multiply(x=w215, y=1.005828380585e-08) -> (x*y=w221:dbl)
        n92 = Divide(x=w221, y=w214) -> (x/y=w220:dbl)
        n93 = Add(x=w219, y=w220) -> (x+y=w208:dbl)
        "Waveform Chart" <- w208
        n94 = Bundle By Name(cluster=w212, "Encoder Data"=w209, "Data Counter"=w206, "First Run"=FALSE, "Yaw"=w208, "TimeStamp Prev"=w217, "Time Delta"=w214) -> (w223:T18)
      }
      frame "Process" {
        n95 = Unbundle By Name(w245) -> ("Yaw"=w242:dbl, "TimeStamp Prev"=w243:dbl, "Time Delta"=w240:dbl, "Data Counter"=w241:u16, "Encoder Data"=w236:T26)
        n96 = Bundle By Name(cluster=T9 {"Yaw"=0.0, "Timestamp"=0.0, "Timestamp Delta"=0.0, "Sample Count"=0} ("element"), "Yaw"=w242, "Timestamp"=w243, "Timestamp Delta"=w240, "Sample Count"=w241) -> (w237:T9)
        n97 = call "Sychronous Odometry Processor.vi"("error in (no error)"=w239, "Encoder Data"=w236, "Heading"=w237) -> ("error out"=w238:errorcluster, "Reset?"=w234:bool)  [unwired: 7 in]
        n98 = case shown="True" w234 {
          tunnel: w245 -> [w247 w250]
          tunnel: [w247 w249] -> w235
          frame False {
          }
          frame True {
            n99 = Bundle By Name(cluster=w250, "Yaw"=0.0) -> (w249:T18)
          }
        }
      }
    }
  }
  n100 = flat-sequence {
    tunnel: w2 -> [w251]
    tunnel: [w251] -> w1
    tunnel: w1 -> [w253]
    frame #0 {
      n101 = Wait (ms)(milliseconds to wait=u32 20000) -> ()  [unwired: 1 out]
    }
    frame #1 {
      n102 = call "ADIS16470 Finish Calibration.vi"("ADIS16470DevRef in"=w253) -> ()  [unwired: 9 in, 2 out]
    }
  }
  n103 = call <vilib>:"NetComm_UsageReport_report.vi"("Instance Number"=u8 1, "Resource Type"=NetComm_UsageReport_ResourceType."ADIS16470") -> ()  [unwired: 10 in]
